vi "SubSystems.vi"(8 "error in":errorcluster) -> ()   [LabVIEW 2018]
doc: "This VI calls the various robot subsystems that will then run in parallel. New subSystems will automatlically script code to make the call."
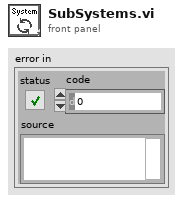
[diagram p1: front panel]
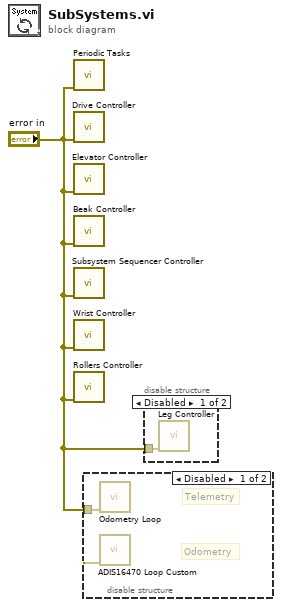
[diagram p0: block diagram]
diagram:
  n1 = call "Periodic Tasks.vi"("error in"="error in") -> ()  [unwired: 1 in, 10 out]
  n2 = call "Drive Controller.vi"("error in"="error in") -> ()  [unwired: 11 in]
  n3 = call "Elevator Controller.vi"("error in"="error in") -> ()  [unwired: 11 in]
  n4 = call "Beak Controller.vi"("error in"="error in") -> ()  [unwired: 11 in]
  n5 = call "Subsystem Sequencer Controller.vi"("error in"="error in") -> ()  [unwired: 11 in]
  n6 = call "Wrist Controller.vi"("error in"="error in") -> ()  [unwired: 11 in]
  n7 = call "Rollers Controller.vi"("error in"="error in") -> ()  [unwired: 11 in]
  n8 = disable-structure shown="Disabled" {
    disable-tunnel: "error in" -> [w2 _]
    frame Disabled {
      # "Odometry"
      # "Telemetry"
      n9 = call "Odometry Loop.vi"("error in (no error)"=w2) -> ()  [unwired: 9 in]
      n10 = call "ADIS16470 Loop Custom.vi"("error in"=w2) -> ()  [unwired: 11 in]
    }
    frame Enabled {
    }
  }
  n11 = disable-structure shown="Disabled" {
    disable-tunnel: "error in" -> [w3 _]
    frame Disabled {
      n12 = call "Leg Controller.vi"("error in"=w3) -> ()  [unwired: 11 in]
    }
    frame Enabled {
    }
  }
